vi "WIP_State_Queue.vi"(8 "error in (no error)":errorcluster, 10 "State In":T1, 11 "Queue In":refnum<queue>) -> (0 "error out":errorcluster, 2 "State Out":T1, 3 "Queue out":refnum<queue>)   [LabVIEW 2020]
uses:
  Controls/WIP_State.ctl
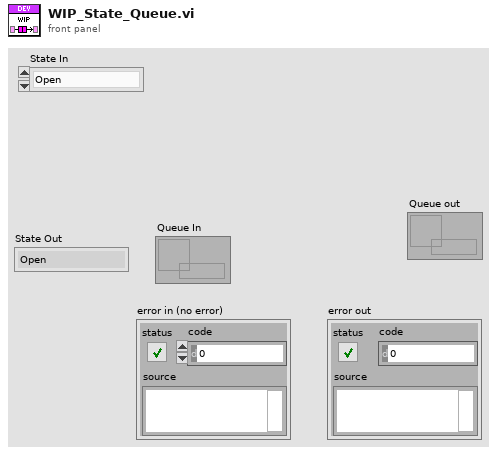
[diagram p1: front panel]
types:
  T1 = typedef "WIP_State.ctl" = enum16{"Open", "Read", "Write", "Read WIP", "Flush", "Close"}
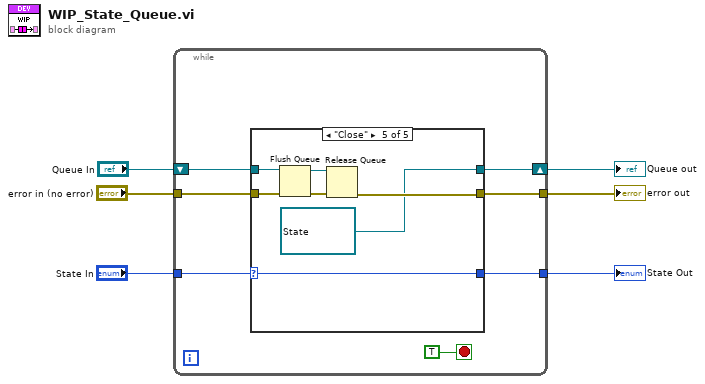
[diagram p0: block diagram]
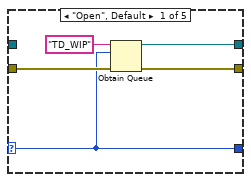
[diagram p2: hidden frame]
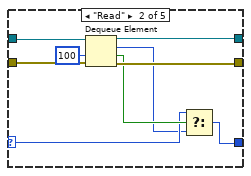
[diagram p3: hidden frame]
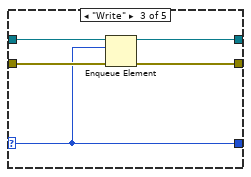
[diagram p4: hidden frame]
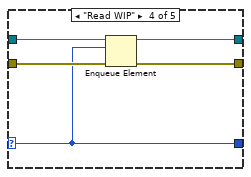
[diagram p5: hidden frame]
diagram:
  n1 = while {
    tunnel: "State In" -> [w9]
    shift-right: [w12] -> w5
    shift-left: "Queue In" -> [w8]
    tunnel: "error in (no error)" -> [w11]
    tunnel: [w13] -> w6
    tunnel: [w7] -> w2
    stop <- TRUE stop-if-true
    n2 = case shown="\"Close\"" w9 {
      selector: w9 -> [w14 w21 w28 w33 w38]
      tunnel: [w18 w24 w29 w34 w40] -> w13
      tunnel: [w17 w23 w30 w35 w39] -> w12
      tunnel: w11 -> [w15 w27 w31 w36 w44]
      tunnel: w8 -> [_ w26 w32 w37 w43]
      tunnel: [w14 w19 w28 w33 w38] -> w7
      frame "Open", Default {
        n3 = Obtain Queue(name (unnamed)="TD_WIP", element data type=w14, error in (no error)=w15) -> (queue out=w17:refnum<queue>, error out=w18:errorcluster)  [unwired: 2 in, 1 out]
      }
      frame "Read" {
        n4 = Dequeue Element(queue=w26, timeout in ms (-1)=100, error in (no error)=w27) -> (queue out=w23:refnum<queue>, element=w20:T1, timed out?=w22:bool, error out=w24:errorcluster)
        n5 = Select(t=w21, s=w22, f=w20) -> (s? t:f=w19:T1)
      }
      frame "Write" {
        n6 = Enqueue Element(queue=w32, element=w28, error in (no error)=w31) -> (queue out=w30:refnum<queue>, error out=w29:errorcluster)  [unwired: 1 in, 1 out]
      }
      frame "Read WIP" {
        n7 = Enqueue Element(queue=w37, element=w33, error in (no error)=w36) -> (queue out=w35:refnum<queue>, error out=w34:errorcluster)  [unwired: 1 in, 1 out]
      }
      frame "Close" {
        w39 = refnum<queue> refnum items=["Open", "Read", "Write", "Read WIP", "Flush", "Close"] ("Queue In")
        n8 = Flush Queue(queue=w43, error in (no error)=w44) -> (queue out=w41:refnum<queue>, error out=w42:errorcluster)  [unwired: 1 out]
        n9 = Release Queue(queue=w41, error in (no error)=w42) -> (error out=w40:errorcluster)  [unwired: 1 in, 2 out]
      }
    }
  }
  "error out" <- w6
  "Queue out" <- w5
  "State Out" <- w2
